vi "Documentation.vi"   [LabVIEW 2019, in "Instrument.Framework-Template.lvclass"]
uses:
  Instrument.Framework-Template.lvclass
  643cabf3-11e0-466e-85d6-f585accee3b6.vi
  bb10f022-7853-4ddd-8dc0-eb6526ad0f54.vi
  61dfef3a-8a93-4f93-91d7-c0ad557d8145.vi
  61dfef3a-8a93-4f93-91d7-c0ad557d8145.vi/a0289200-95e1-4249-98a2-0a47764017b7.vi
  61dfef3a-8a93-4f93-91d7-c0ad557d8145.vi/ef93eee4-b3f8-407d-be7e-7b70ab04c88e.vi
  <vilib>/Utility/Data Type/Get Numeric Information.vi
  <userlib>/LevyLab/Instrument Framework/Instrument/API/Instrument.sendMessageToProcess (string).vi
  <vilib>/Utility/Data Type/Get Type Information.vi
  <vilib>/JDP Science/JSONtext/JSON text to Variant.vi
  <userlib>/LevyLab/Instrument Framework/Instrument/Instrument.lvclass
  <vilib>/JKI/JKI SMO/SMO/SMO.lvclass
  <userlib>/LevyLab/Instrument Framework/Instrument/Typedefs/Instrument.ProtectedCommands--Enum.ctl
  Typedefs/Instrument.Framework-Template.PublicCommands--Enum.ctl
  <userlib>/LevyLab/Instrument Framework/Instrument/Typedefs/Instrument.Commands--Enum.ctl
  Typedefs/Instrument.Framework-Template.getAll--Cluster.ctl
  Typedefs/Instrument.Framework-Template.Configuration--Cluster.ctl
  Typedefs/Instrument.Framework-Template.ProtectedCommands--Enum.ctl
  <vilib>/JDP Science/JSONtext/LVClass Serializer/JSONtext LVClass Serializer.lvclass
  Instrument UI.Framework-Template/Instrument UI.Framework-Template.lvclass
  Instrument UI.Framework-Template/Instrument UI.Framework-Template.UI--Cluster.ctl
  <userlib>/LevyLab/Instrument Framework/Instrument Types/Amplifier/Instrument.Amplifier.lvclass
  <userlib>/LevyLab/Instrument Framework/Instrument Types/CBridge/Instrument.CBridge.lvclass
  <userlib>/LevyLab/Instrument Framework/Instrument Types/Cryostat/Instrument.Cryostat.lvclass
  <userlib>/LevyLab/Instrument Framework/Instrument Types/Delay Line/Instrument.DelayLine.lvclass
  <userlib>/LevyLab/Instrument Framework/Instrument Types/Lockin/Instrument.LockinAPI.lvclass
  <userlib>/LevyLab/Instrument Framework/Instrument Types/Strain/Instrument.Strain.lvclass
  <userlib>/LevyLab/Instrument Framework/Instrument Types/VNA/Instrument.VNA.lvclass
  <userlib>/LevyLab/Instrument Framework/Instrument Types/SCPI/Instrument.SCPI.lvclass
  <userlib>/LevyLab/Instrument Framework/Instrument Types/SignalGenerator/Instrument.SignalGenerator.lvclass
  <userlib>/LevyLab/Instrument Framework/Instrument Types/VSource/Instrument.VSource.lvclass
  <userlib>/LevyLab/Instrument Framework/Instrument UI/Instrument UI.lvclass
  <vilib>/JKI/JKI SMO/SMO.UI/SMO.UI.lvclass
  C:/Program Files (x86)/National Instruments/LabVIEW 2019/user.lib/LevyLab/Instrument Framework/Instrument Types/SCPI/Instrument.SCPI.lvclass
  C:/Program Files (x86)/National Instruments/LabVIEW 2019/user.lib/LevyLab/Instrument Framework/Instrument/Instrument.lvclass
  C:/Program Files (x86)/National Instruments/LabVIEW 2019/vi.lib/JKI/JKI SMO/SMO/SMO.lvclass
  C:/Program Files (x86)/National Instruments/LabVIEW 2019/user.lib/LevyLab/Instrument Framework/Instrument UI/Instrument UI.lvclass
  C:/Program Files (x86)/National Instruments/LabVIEW 2019/vi.lib/JKI/JKI SMO/SMO.UI/SMO.UI.lvclass
types:
  T1 = typedef "Instrument.Framework-Template.lvclass/Instrument.Framework-Template.Configuration--Cluster.ctl" = cluster{"Example Setting 1":dbl, "Example Setting 2":dbl, "Example Setting 3":string}
  T2 = typedef "Instrument.Framework-Template.lvclass/Instrument.Framework-Template.getAll--Cluster.ctl" = cluster{"Levy 1":dbl, "Logger SMO":dbl, "SMO Boolean":bool, "SMO String":string}
  T3 = typedef "Instrument.Framework-Template.lvclass/Instrument.Framework-Template.ProtectedCommands--Enum.ctl" = enum16{"doProtected"}
  T4 = typedef "Instrument.Framework-Template.lvclass/Instrument.Framework-Template.PublicCommands--Enum.ctl" = enum16{"doSomething"}
  T5 = typedef "Instrument.lvclass/Instrument.Commands--Enum.ctl" = enum16{"ACK", "HELP", "IDN", "getAll", "getAllData"}
  T6 = typedef "Instrument.lvclass/Instrument.ProtectedCommands--Enum.ctl" = enum16{"setConfiguration", "setLogData", "setIDN", "setAll", "setAllData"}
  T7 = typedef "Instrument UI.Framework-Template.lvclass/Instrument UI.Framework-Template.UI--Cluster.ctl" = cluster{"Parameter":dbl, "Parameter 2":string}
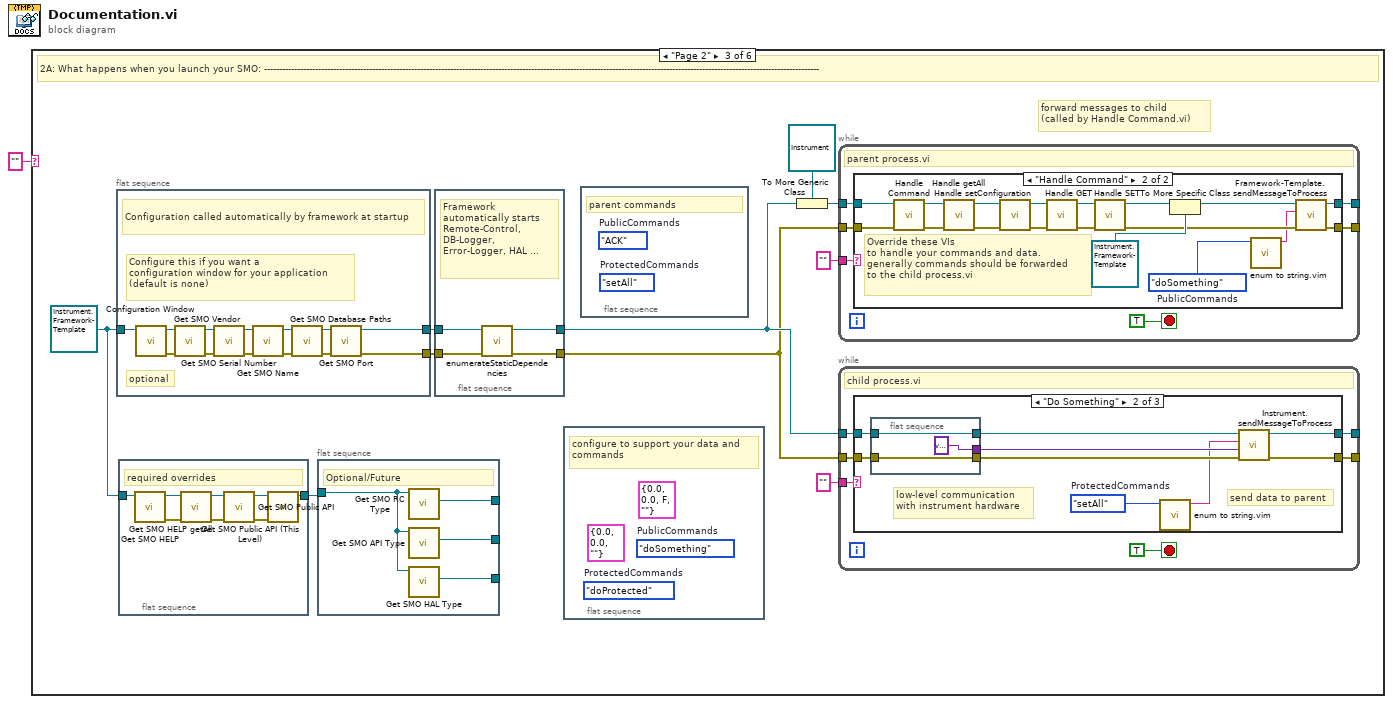
[diagram p0: block diagram]
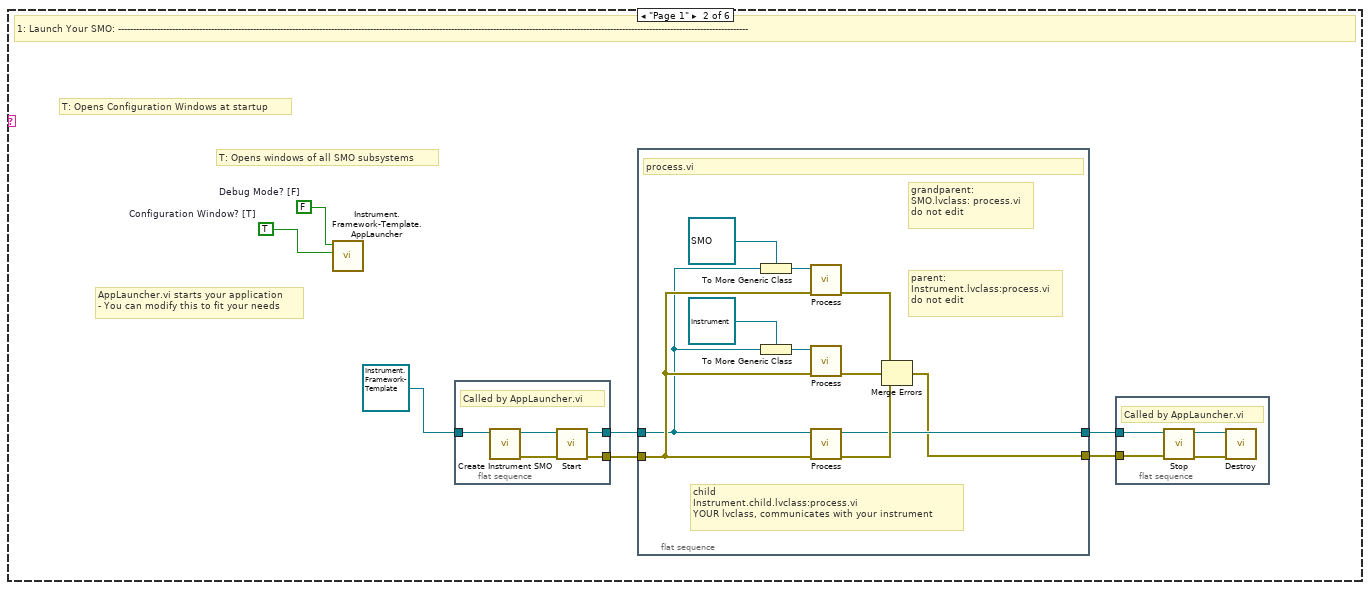
[diagram p3: hidden frame]
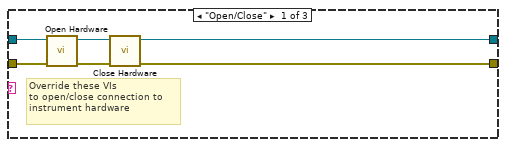
[diagram p4: hidden frame]
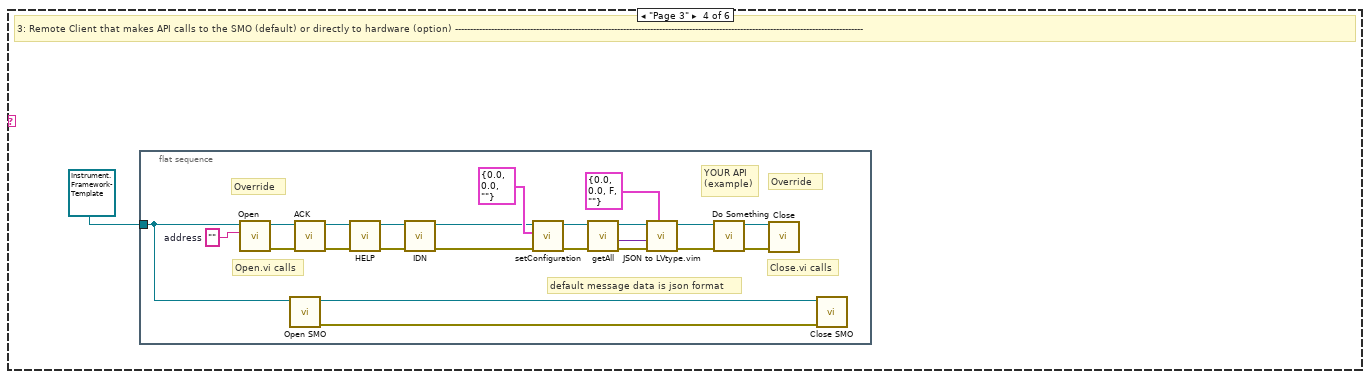
[diagram p7: hidden frame]
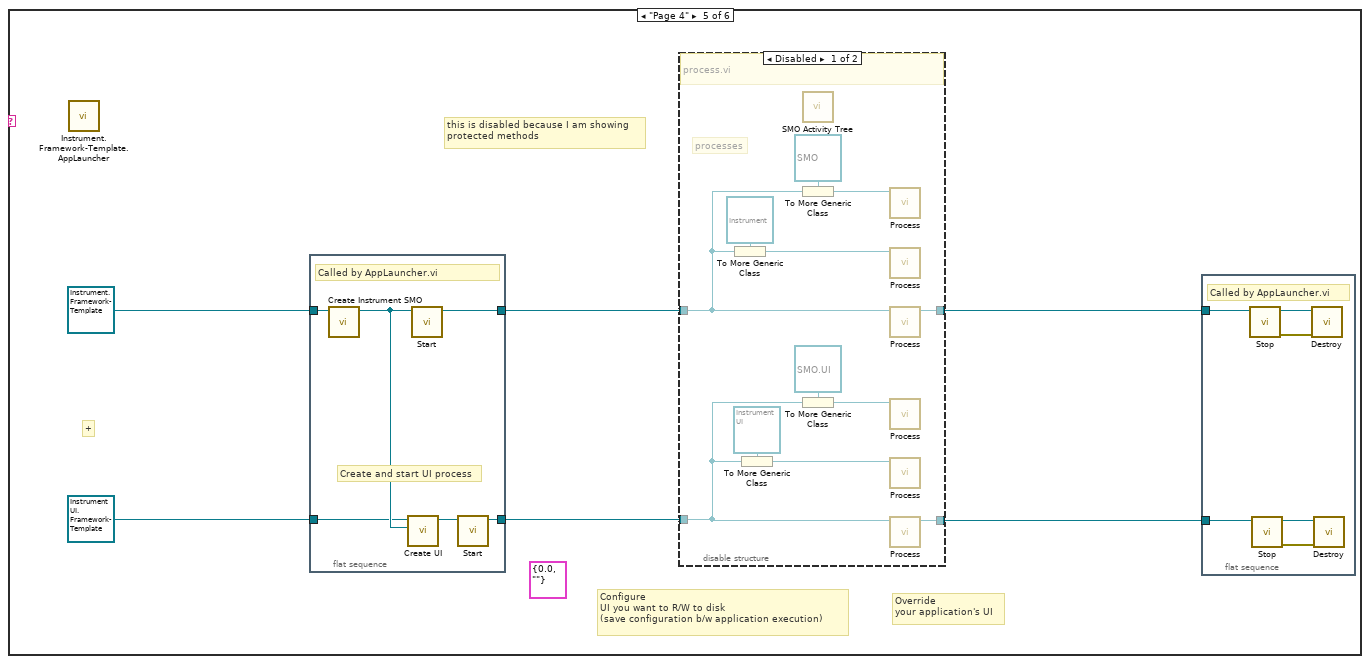
[diagram p8: hidden frame]
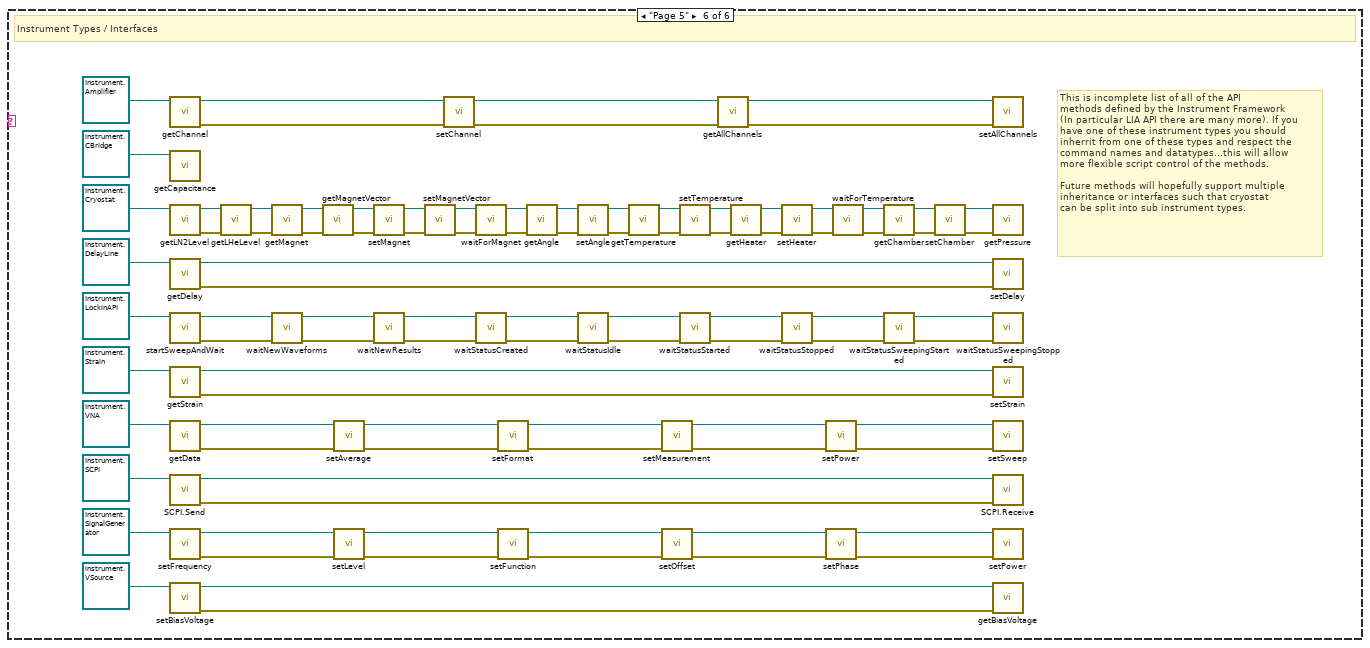
[diagram p10: hidden frame]
diagram:
  n1 = case shown="\"Page 2\"" "" {
    frame Default {
    }
    frame "Page 1" {
      w7 = TRUE  # Configuration Window? [T]
      w8 = FALSE  # Debug Mode? [F]
      # "AppLauncher.vi starts your application\n- You can modify this to fit your needs"
      # "T: Opens windows of all SMO subsystems"
      # "T: Opens Configuration Windows at startup"
      # "1: Launch Your SMO: ------------------------------------------------------------------------------------------------------------------------------------------------------------------------------------------------------------------"
      n2 = call "Instrument.Framework-Template.AppLauncher.vi"("Config Window"=w7, "Debug Mode"=w8) -> ()  [unwired: 9 in, 1 out]
      n3 = flat-sequence {
        tunnel: [w26] -> w3
        tunnel: [w25] -> w5
        tunnel: refnum<class "Instrument.Framework-Template.lvclass"> refnum ("Instrument.Template.lvclass") -> [w24]
        frame #0 {
          # "Called by AppLauncher.vi"
          n4 = call <userlib>:"Create Instrument SMO.vi"("Instrument in"=w24) -> ("error out"=w27:errorcluster, "Instrument out"=w28:refnum<class "Instrument.Framework-Template.lvclass">)  [unwired: 9 in]
          n5 = call <vilib>:"Start.vi"("error in (no error)"=w27, "SMO"=w28) -> ("error out"=w25:errorcluster, "SMO out"=w26:refnum<class "Instrument.Framework-Template.lvclass">)  [unwired: 8 in]
        }
      }
      n6 = flat-sequence {
        tunnel: [w10] -> w6
        tunnel: w5 -> [w18]
        tunnel: [w13] -> w4
        tunnel: w3 -> [w12]
        frame #0 {
          # "child\nInstrument.child.lvclass:process.vi\nYOUR lvclass, communicates with your instrument"
          # "grandparent:\nSMO.lvclass: process.vi\ndo not edit"
          # "parent:\nInstrument.lvclass:process.vi\ndo not edit"
          # "process.vi"
          n7 = To More Generic Class(target class=refnum<class "SMO.lvclass"> refnum ("SMO"), reference=w12) -> (generic class reference=w19:refnum<class "SMO.lvclass">)
          n8 = To More Generic Class(target class=refnum<class "Instrument.lvclass"> refnum ("Instrument"), reference=w12) -> (generic class reference=w17:refnum<class "Instrument.lvclass">)
          n9 = call-dynamic "Process.vi"("error in"=w18, "SMO"=w19) -> ("error out"=w14:errorcluster)  [unwired: 8 in, 1 out]
          n10 = call-dynamic "Process.vi"("error in"=w18, "Instrument"=w17) -> ("error out"=w16:errorcluster)  [unwired: 8 in, 1 out]
          n11 = call-dynamic "Process.vi"("error in"=w18, "Instrument.Framework-Template in"=w12) -> ("error out"=w15:errorcluster, "Instrument.Framework-Template out"=w13:refnum<class "Instrument.Framework-Template.lvclass">)  [unwired: 8 in]
          n12 = Merge Errors(w14, w16, w15) -> (w10:errorcluster)
        }
      }
      n13 = flat-sequence {
        tunnel: w4 -> [w21]
        tunnel: w6 -> [w20]
        frame #0 {
          # "Called by AppLauncher.vi"
          n14 = call <vilib>:"Stop.vi"("error in (no error)"=w20, "SMO"=w21) -> ("error out"=w23:errorcluster, "SMO out"=w22:refnum<class "Instrument.Framework-Template.lvclass">)  [unwired: 8 in]
          n15 = call <vilib>:"Destroy.vi"("error in (no error)"=w23, "SMO"=w22) -> ()  [unwired: 9 in, 1 out]
        }
      }
    }
    frame "Page 2" {
      w32 = refnum<class "Instrument.Framework-Template.lvclass"> refnum ("Instrument.Template.lvclass")
      # "forward messages to child\n(called by Handle Command.vi)"
      # "2A: What happens when you launch your SMO: -----------------------------------------------------------------------------------------------------------------------------------------------------------------------------------------"
      n16 = flat-sequence {
        tunnel: w32 -> [w61]
        tunnel: [w51] -> w33
        tunnel: [w52] -> w34
        frame #0 {
          # "optional"
          # "Configure this if you want a\nconfiguration window for your application\n(default is none)"
          # "Configuration called automatically by framework at startup"
          n17 = call-dynamic "Configuration Window.vi"("Example Instrument in"=w61) -> ("error out"=w63:errorcluster, "Example Instrument out"=w62:refnum<class "Instrument.Framework-Template.lvclass">)  [unwired: 9 in]
          n18 = call-dynamic "Get SMO Vendor.vi"("error in (no error)"=w63, "Instrument.Framework-Template in"=w62) -> ("error out"=w53:errorcluster, "Instrument.Framework-Template out"=w58:refnum<class "Instrument.Framework-Template.lvclass">)  [unwired: 7 in, 1 out]
          n19 = call-dynamic "Get SMO Serial Number.vi"("error in (no error)"=w53, "Instrument.Framework-Template in"=w58) -> ("error out"=w54:errorcluster, "Instrument.Framework-Template out"=w57:refnum<class "Instrument.Framework-Template.lvclass">)  [unwired: 7 in, 1 out]
          n20 = call-dynamic "Get SMO Name.vi"("error in (no error)"=w54, "Instrument.Framework-Template in"=w57) -> ("error out"=w55:errorcluster, "Instrument.Framework-Template out"=w56:refnum<class "Instrument.Framework-Template.lvclass">)  [unwired: 7 in, 1 out]
          n21 = call-dynamic "Get SMO Database Paths.vi"("error in (no error)"=w55, "Instrument.Framework-Template in"=w56) -> ("error out"=w59:errorcluster, "Instrument.Framework-Template out"=w60:refnum<class "Instrument.Framework-Template.lvclass">)  [unwired: 7 in, 1 out]
          n22 = call-dynamic "Get SMO Port.vi"("error in (no error)"=w59, "Instrument.Framework-Template in"=w60) -> ("error out"=w51:errorcluster, "Instrument.Framework-Template out"=w52:refnum<class "Instrument.Framework-Template.lvclass">)  [unwired: 7 in, 1 out]
        }
      }
      n23 = flat-sequence {
        tunnel: w32 -> [w40]
        tunnel: [w39] -> w31
        frame #0 {
          # "required overrides"
          n24 = call-dynamic "Get SMO HELP.vi"("Instrument.Framework-Template in"=w40) -> ("error out"=w46:errorcluster, "Instrument.Framework-Template out"=w45:refnum<class "Instrument.Framework-Template.lvclass">)  [unwired: 8 in, 1 out]
          n25 = call-dynamic "Get SMO HELP getAll.vi"("error in (no error)"=w46, "Instrument.Framework-Template in"=w45) -> ("error out"=w43:errorcluster, "Instrument.Framework-Template out"=w44:refnum<class "Instrument.Framework-Template.lvclass">)  [unwired: 6 in, 2 out]
          n26 = call-dynamic "Get SMO Public API.vi"("error in (no error)"=w43, "Instrument.Framework-Template in"=w44) -> ("error out"=w42:errorcluster, "Instrument.Framework-Template out"=w41:refnum<class "Instrument.Framework-Template.lvclass">)  [unwired: 7 in, 1 out]
          n27 = call-dynamic "Get SMO Public API (This Level).vi"("error in (no error)"=w42, "Instrument.Framework-Template in"=w41) -> ("Instrument.Framework-Template out"=w39:refnum<class "Instrument.Framework-Template.lvclass">)  [unwired: 7 in, 2 out]
        }
      }
      n28 = flat-sequence {
        tunnel: w31 -> [w67]
        tunnel: [w66] -> _
        tunnel: [w65] -> _
        tunnel: [w64] -> _
        frame #0 {
          # "Optional/Future"
          n29 = call-dynamic "Get SMO RC Type.vi"("Instrument in"=w67) -> ("RemoteControl"=w66:refnum<class "RemoteControl.lvclass">)  [unwired: 8 in, 2 out]
          n30 = call-dynamic "Get SMO API Type.vi"("Instrument in"=w67) -> ("API"=w65:refnum<class "API.lvclass">)  [unwired: 8 in, 2 out]
          n31 = call-dynamic "Get SMO HAL Type.vi"("Instrument in"=w67) -> ("Dependencies.HAL"=w64:refnum<class "HAL.lvclass">)  [unwired: 8 in, 2 out]
        }
      }
      n32 = flat-sequence {
        tunnel: w34 -> [w50]
        tunnel: w33 -> [w49]
        tunnel: [w48] -> w30
        tunnel: [w47] -> w29
        frame #0 {
          # "Framework automatically starts\nRemote-Control, DB-Logger, Error-Logger, HAL ..."
          n33 = call-dynamic "enumerateStaticDependencies.vi"("error in (no error)"=w49, "Instrument"=w50) -> ("error out"=w47:errorcluster, "Instrument out"=w48:refnum<class "Instrument.Framework-Template.lvclass">)  [unwired: 7 in, 1 out]
        }
      }
      n34 = flat-sequence {
        frame #0 {
          (unwired) Instrument.Framework-Template.ProtectedCommands--Enum."doProtected"  # ProtectedCommands
          (unwired) T1 {"Example Setting 1"=0.0, "Example Setting 2"=0.0, "Example Setting 3"=""} ("Configuration")
          (unwired) T2 {"Levy 1"=0.0, "Logger SMO"=0.0, "SMO Boolean"=FALSE, "SMO String"=""} ("getAll")
          (unwired) Instrument.Framework-Template.PublicCommands--Enum."doSomething"  # PublicCommands
          # "configure to support your data and commands"
        }
      }
      n35 = flat-sequence {
        frame #0 {
          (unwired) Instrument.Commands--Enum."ACK"  # PublicCommands
          (unwired) Instrument.ProtectedCommands--Enum."setAll"  # ProtectedCommands
          # "parent commands"
        }
      }
      n36 = To More Generic Class(target class=refnum<class "Instrument.lvclass"> refnum ("Instrument"), reference=w30) -> (generic class reference=w35:refnum<class "Instrument.lvclass">)
      n37 = while {
        tunnel: "" -> [w99]
        tunnel: w35 -> [w97]
        tunnel: [w96] -> _
        tunnel: w29 -> [w95]
        tunnel: [w94] -> _
        stop <- TRUE stop-if-true
        # "parent process.vi"
        n38 = case shown="\"Handle Command\"" w99 {
          tunnel: w97 -> [w101 w119]
          tunnel: [w101 w113] -> w96
          tunnel: w95 -> [w100 w118]
          tunnel: [w100 w112] -> w94
          frame Default {
          }
          frame "Handle Command" {
            w103 = Instrument.Framework-Template.PublicCommands--Enum."doSomething"  # PublicCommands
            # "Override these VIs\nto handle your commands and data.\ngenerally commands should be forwarded\nto the child process.vi"
            n39 = call-dynamic "Handle Command.vi"("error in (no error)"=w118, "Instrument in"=w119) -> ("error out"=w114:errorcluster, "Instrument out"=w117:refnum<class "Instrument.lvclass">)  [unwired: 6 in, 2 out]
            n40 = call-dynamic "Handle getAll.vi"("error in (no error)"=w114, "Instrument in"=w117) -> ("error out"=w115:errorcluster, "Instrument out"=w116:refnum<class "Instrument.lvclass">)  [unwired: 7 in, 1 out]
            n41 = call-dynamic "Handle setConfiguration.vi"("error in (no error)"=w115, "Instrument in"=w116) -> ("error out"=w108:errorcluster, "Instrument out"=w109:refnum<class "Instrument.lvclass">)  [unwired: 8 in]
            n42 = call-dynamic "Handle GET.vi"("error in (no error)"=w108, "Instrument in"=w109) -> ("error out"=w106:errorcluster, "Instrument out"=w107:refnum<class "Instrument.lvclass">)  [unwired: 7 in, 1 out]
            n43 = call-dynamic "Handle SET.vi"("error in (no error)"=w106, "Instrument in"=w107) -> ("error out"=w104:errorcluster, "Instrument out"=w105:refnum<class "Instrument.lvclass">)  [unwired: 7 in, 1 out]
            n44 = To More Specific Class(target class=refnum<class "Instrument.Framework-Template.lvclass"> refnum ("Instrument.Template.lvclass"), reference=w105) -> (specific class reference=w111:refnum<class "Instrument.Framework-Template.lvclass">)  [unwired: 1 in, 1 out]
            n45 = call "enum to string.vim"("enum in"=w103) -> ("string out"=w102:string)  [unwired: 9 in, 1 out]
            n46 = call "Framework-Template.sendMessageToProcess.vi"("error in (no error)"=w104, "Command"=w102, "Instrument.Framework-Template in"=w111) -> ("error out"=w112:errorcluster, "Instrument.Framework-Template out"=w113:refnum<class "Instrument.Framework-Template.lvclass">)  [unwired: 7 in]
          }
        }
      }
      n47 = while {
        tunnel: "" -> [w73]
        tunnel: w30 -> [w71]
        tunnel: [w70] -> _
        tunnel: w29 -> [w69]
        tunnel: [w68] -> _
        stop <- TRUE stop-if-true
        # "child process.vi"
        n48 = case shown="\"Do Something\"" w73 {
          tunnel: w71 -> [w76 w84 w93]
          tunnel: [w75 w88 w93] -> w70
          tunnel: w69 -> [w79 w86 w92]
          tunnel: [w74 w87 w92] -> w68
          frame "Open/Close" {
            # "Override these VIs\nto open/close connection to\ninstrument hardware"
            n49 = call-dynamic "Open Hardware.vi"("error in (no error)"=w79, "Instrument in"=w76) -> ("error out"=w78:errorcluster, "Instrument out"=w77:refnum<class "Instrument.Framework-Template.lvclass">)  [unwired: 8 in]
            n50 = call-dynamic "Close Hardware.vi"("error in (no error)"=w78, "Instrument in"=w77) -> ("error out"=w74:errorcluster, "Instrument out"=w75:refnum<class "Instrument.Framework-Template.lvclass">)  [unwired: 8 in]
          }
          frame "Do Something" {
            w81 = Instrument.ProtectedCommands--Enum."setAll"  # ProtectedCommands
            # "low-level communication\nwith instrument hardware"
            # "send data to parent"
            n51 = flat-sequence {
              tunnel: w86 -> [w91]
              tunnel: [w91] -> w85
              tunnel: w84 -> [w90]
              tunnel: [w90] -> w83
              tunnel: [variant ("Data")] -> w82
              frame #0 {
              }
            }
            n52 = call "enum to string.vim"("enum in"=w81) -> ("string out"=w80:string)  [unwired: 9 in, 1 out]
            n53 = call-poly <userlib>:"Instrument.sendMessageToProcess.vi"("error in (no error)"=w85, "Data"=w82, "Command"=w80, "Instrument"=w83) -> ("error out"=w87:errorcluster, "Instrument out"=w88:refnum<class "Instrument.Framework-Template.lvclass">)  [unwired: 6 in]
          }
          frame Default {
          }
        }
      }
    }
    frame "Page 3" {
      # "3: Remote Client that makes API calls to the SMO (default) or directly to hardware (option) ----------------------------------------------------------------------------------------------------------------------------------------"
      n54 = flat-sequence {
        tunnel: refnum<class "Instrument.Framework-Template.lvclass"> refnum ("Instrument.Template.lvclass") -> [w130]
        frame #0 {
          w133 = ""  # address
          # "default message data is json format"
          # "Close.vi calls"
          # "Open.vi calls"
          # "YOUR API\n(example)"
          # "Override"
          # "Override"
          n55 = call-dynamic "Open.vi"("address"=w133, "Instrument.Framework-Template in"=w130) -> ("error out"=w142:errorcluster, "Instrument.Framework-Template out"=w141:refnum<class "Instrument.Framework-Template.lvclass">)  [unwired: 8 in]
          n56 = call <userlib>:"Open SMO.vi"("Instrument in"=w130) -> ("error out"=w131:errorcluster, "Instrument out"=w132:refnum<class "Instrument.Framework-Template.lvclass">)  [unwired: 9 in]
          n57 = call <userlib>:"ACK.vi"("error in (no error)"=w142, "Instrument in"=w141) -> ("error out"=w140:errorcluster, "Instrument out"=w139:refnum<class "Instrument.Framework-Template.lvclass">)  [unwired: 7 in, 1 out]
          n58 = call <userlib>:"HELP.vi"("error in (no error)"=w140, "Instrument in"=w139) -> ("error out"=w123:errorcluster, "Instrument in"=w124:refnum<class "Instrument.Framework-Template.lvclass">)  [unwired: 7 in, 1 out]
          n59 = call <userlib>:"IDN.vi"("error in (no error)"=w123, "Instrument in"=w124) -> ("error out"=w121:errorcluster, "Instrument in"=w122:refnum<class "Instrument.Framework-Template.lvclass">)  [unwired: 7 in, 1 out]
          n60 = call <userlib>:"setConfiguration.vi"("error in (no error)"=w121, "Configuration"=T1 {"Example Setting 1"=0.0, "Example Setting 2"=0.0, "Example Setting 3"=""}, "Instrument in"=w122) -> ("error out"=w134:errorcluster, "Instrument out"=w135:refnum<class "Instrument.Framework-Template.lvclass">)  [unwired: 7 in]
          n61 = call <userlib>:"getAll.vi"("error in (no error)"=w134, "Instrument in"=w135) -> ("error out"=w129:errorcluster, "getAll"=w125:variant, "Instrument out"=w126:refnum<class "Instrument.Framework-Template.lvclass">)  [unwired: 7 in]
          n62 = call "JSON to LVtype.vim"("type"=T2 {"Levy 1"=0.0, "Logger SMO"=0.0, "SMO Boolean"=FALSE, "SMO String"=""} ("getAll"), "error in (no error)"=w129, "JSON Data in"=w125) -> ("error out"=w127:errorcluster)  [unwired: 7 in, 1 out]
          n63 = call-dynamic "Do Something.vi"("error in (no error)"=w127, "Instrument.Framework-Template in"=w126) -> ("error out"=w137:errorcluster, "Instrument.Framework-Template out"=w138:refnum<class "Instrument.Framework-Template.lvclass">)  [unwired: 8 in]
          n64 = call-dynamic "Close.vi"("error in (no error)"=w137, "Instrument.Framework-Template in"=w138) -> ()  [unwired: 8 in, 2 out]
          n65 = call <userlib>:"Close SMO.vi"("error in (no error)"=w131, "Instrument in"=w132) -> ()  [unwired: 8 in, 2 out]
        }
      }
    }
    frame "Page 4" {
      (unwired) T7 {"Parameter"=0.0, "Parameter 2"=""} ("UI")
      # "this is disabled because I am showing\nprotected methods"
      # "Configure\nUI you want to R/W to disk\n(save configuration b/w application execution)"
      # "Override\nyour application's UI"
      # "+"
      n66 = call "Instrument.Framework-Template.AppLauncher.vi"() -> ()  [unwired: 11 in, 1 out]
      n67 = flat-sequence {
        tunnel: [w160] -> w146
        tunnel: refnum<class "Instrument.Framework-Template.lvclass"> refnum ("Instrument.Template.lvclass") -> [w159]
        tunnel: refnum<class "Instrument UI.Framework-Template.lvclass"> refnum ("Instrument UI.Template.lvclass") -> [w157]
        tunnel: [w155] -> w144
        frame #0 {
          # "Create and start UI process"
          # "Called by AppLauncher.vi"
          n68 = call <userlib>:"Create Instrument SMO.vi"("Instrument in"=w159) -> ("Instrument out"=w158:refnum<class "Instrument.Framework-Template.lvclass">)  [unwired: 9 in, 1 out]
          n69 = call <userlib>:"Create UI.vi"("Instrument in"=w158, "Instrument UI"=w157) -> ("Instrument UI out"=w156:refnum<class "Instrument UI.Framework-Template.lvclass">)  [unwired: 8 in, 1 out]
          n70 = call <vilib>:"Start.vi"("SMO"=w158) -> ("SMO out"=w160:refnum<class "Instrument.Framework-Template.lvclass">)  [unwired: 9 in, 1 out]
          n71 = call <vilib>:"Start.vi"("SMO"=w156) -> ("SMO out"=w155:refnum<class "Instrument UI.Framework-Template.lvclass">)  [unwired: 9 in, 1 out]
        }
      }
      n72 = disable-structure shown="Disabled" {
        disable-tunnel: [w172 w174] -> w147
        disable-tunnel: w146 -> [w171 w174]
        disable-tunnel: w144 -> [w170 w173]
        disable-tunnel: [w169 w173] -> w143
        frame Disabled {
          # "processes"
          # "process.vi"
          n73 = To More Generic Class(target class=refnum<class "Instrument.lvclass"> refnum ("Instrument"), reference=w171) -> (generic class reference=w167:refnum<class "Instrument.lvclass">)
          n74 = To More Generic Class(target class=refnum<class "Instrument UI.lvclass"> refnum ("Instrument UI"), reference=w170) -> (generic class reference=w163:refnum<class "Instrument UI.lvclass">)
          n75 = call <vilib>:"SMO Activity Tree.vi"() -> ()  [unwired: 12 in]
          n76 = To More Generic Class(target class=refnum<class "SMO.lvclass"> refnum ("SMO"), reference=w171) -> (generic class reference=w168:refnum<class "SMO.lvclass">)
          n77 = To More Generic Class(target class=refnum<class "SMO.UI.lvclass"> refnum ("SMO.UI"), reference=w170) -> (generic class reference=w161:refnum<class "SMO.UI.lvclass">)
          n78 = call-dynamic "Process.vi"("SMO"=w168) -> ()  [unwired: 9 in, 2 out]
          n79 = call-dynamic "Process.vi"("Instrument"=w167) -> ()  [unwired: 9 in, 2 out]
          n80 = call-dynamic "Process.vi"("Instrument.Framework-Template in"=w171) -> ("Instrument.Framework-Template out"=w172:refnum<class "Instrument.Framework-Template.lvclass">)  [unwired: 9 in, 1 out]
          n81 = call-dynamic "Process.vi"("SMO.UI"=w161) -> ()  [unwired: 9 in, 2 out]
          n82 = call-dynamic "Process.vi"("Instrument UI in"=w163) -> ()  [unwired: 9 in, 2 out]
          n83 = call-dynamic "Process.vi"("Instrument UI.Framework-Template"=w170) -> ("Instrument UI.Framework-Template out"=w169:refnum<class "Instrument UI.Framework-Template.lvclass">)  [unwired: 9 in, 1 out]
        }
        frame Enabled {
        }
      }
      n84 = flat-sequence {
        tunnel: w147 -> [w152]
        tunnel: w143 -> [w150]
        frame #0 {
          # "Called by AppLauncher.vi"
          n85 = call <vilib>:"Stop.vi"("SMO"=w152) -> ("error out"=w154:errorcluster, "SMO out"=w153:refnum<class "Instrument.Framework-Template.lvclass">)  [unwired: 9 in]
          n86 = call <vilib>:"Stop.vi"("SMO"=w150) -> ("error out"=w151:errorcluster, "SMO out"=w149:refnum<class "Instrument UI.Framework-Template.lvclass">)  [unwired: 9 in]
          n87 = call <vilib>:"Destroy.vi"("error in (no error)"=w154, "SMO"=w153) -> ()  [unwired: 9 in, 1 out]
          n88 = call <vilib>:"Destroy.vi"("error in (no error)"=w151, "SMO"=w149) -> ()  [unwired: 9 in, 1 out]
        }
      }
    }
    frame "Page 5" {
      # "This is incomplete list of all of the API\nmethods defined by the Instrument Framework\n(In particular LIA API there are many more). If you\nhave one of these instrument types you should\ninherrit from one of these types and respect the \ncommand names and datatypes...this will allow\nmore flexible script control of the methods.\n\nFuture methods will hopefully support multiple\ninheritance or interfaces such that cryostat\ncan be split into sub instrument types."
      # "Instrument Types / Interfaces"
      n89 = call-dynamic "getChannel.vi"("Instrument.Amplifier in"=refnum<class "Instrument.Amplifier.lvclass"> refnum ("Instrument.Amplifier.lvclass")) -> ("error out"=w255:errorcluster, "Instrument.Amplifier out"=w256:refnum<class "Instrument.Amplifier.lvclass">)  [unwired: 8 in, 1 out]
      n90 = call-dynamic "getCapacitance.vi"("Instrument.CBridge in"=refnum<class "Instrument.CBridge.lvclass"> refnum ("Instrument.CBridge.lvclass")) -> ()  [unwired: 8 in, 3 out]
      n91 = call-dynamic "getLN2Level.vi"("Instrument.Cryostat in"=refnum<class "Instrument.Cryostat.lvclass"> refnum ("Instrument.Cryostat.lvclass")) -> ("error out"=w249:errorcluster, "Instrument.Cryostat out"=w250:refnum<class "Instrument.Cryostat.lvclass">)  [unwired: 8 in, 1 out]
      n92 = call <userlib>:"getDelay.vi"("Instrument.DelayLine in"=refnum<class "Instrument.DelayLine.lvclass"> refnum ("Instrument.DelayLine.lvclass")) -> ("error out"=w217:errorcluster, "Instrument.DelayLine out"=w218:refnum<class "Instrument.DelayLine.lvclass">)  [unwired: 7 in, 2 out]
      n93 = call-dynamic "startSweepAndWait.vi"("Instrument.LockinAPI in"=refnum<class "Instrument.LockinAPI.lvclass"> refnum ("Instrument.LockinAPI.lvclass")) -> ("error out"=w215:errorcluster, "Instrument.LockinAPI out"=w216:refnum<class "Instrument.LockinAPI.lvclass">)  [unwired: 9 in]
      n94 = call-dynamic "getStrain.vi"("Instrument.Strain in"=refnum<class "Instrument.Strain.lvclass"> refnum ("Instrument.Strain.lvclass")) -> ("error out"=w199:errorcluster, "Instrument.Strain out"=w200:refnum<class "Instrument.Strain.lvclass">)  [unwired: 8 in, 1 out]
      n95 = call-dynamic "getData.vi"("Instrument.VSource in"=refnum<class "Instrument.VNA.lvclass"> refnum ("Instrument.VNA.lvclass")) -> ("error out"=w197:errorcluster, "Instrument.VSource out"=w198:refnum<class "Instrument.VNA.lvclass">)  [unwired: 8 in, 1 out]
      n96 = call-dynamic "SCPI.Send.vi"("Instrument.SCPI in"=refnum<class "Instrument.SCPI.lvclass"> refnum ("Instrument.SCPI.lvclass")) -> ("error out"=w187:errorcluster, "Instrument.SCPI out"=w188:refnum<class "Instrument.SCPI.lvclass">)  [unwired: 9 in]
      n97 = call-dynamic "setFrequency.vi"("Instrument.SignalGenerator in"=refnum<class "Instrument.SignalGenerator.lvclass"> refnum ("Instrument.SignalGenerator.lvclass")) -> ("error out"=w185:errorcluster, "Instrument.SignalGenerator out"=w186:refnum<class "Instrument.SignalGenerator.lvclass">)  [unwired: 9 in]
      n98 = call-dynamic "setBiasVoltage.vi"("Instrument.VSource in"=refnum<class "Instrument.VSource.lvclass"> refnum ("Instrument.VSource.lvclass")) -> ("error out"=w175:errorcluster, "Instrument.VSource out"=w176:refnum<class "Instrument.VSource.lvclass">)  [unwired: 9 in]
      n99 = call-dynamic "getLHeLevel.vi"("error in (no error)"=w249, "Instrument.Cryostat in"=w250) -> ("error out"=w247:errorcluster, "Instrument.Cryostat out"=w248:refnum<class "Instrument.Cryostat.lvclass">)  [unwired: 7 in, 1 out]
      n100 = call-dynamic "getMagnet.vi"("error in (no error)"=w247, "Instrument.Cryostat in"=w248) -> ("error out"=w245:errorcluster, "Instrument.Cryostat out"=w246:refnum<class "Instrument.Cryostat.lvclass">)  [unwired: 5 in, 3 out]
      n101 = call-dynamic "waitNewWaveforms.vi"("error in (no error)"=w215, "Instrument.LockinAPI in"=w216) -> ("error out"=w213:errorcluster, "Instrument.LockinAPI out"=w214:refnum<class "Instrument.LockinAPI.lvclass">)  [unwired: 7 in, 1 out]
      n102 = call-dynamic "getMagnetVector.vi"("error in (no error)"=w245, "Instrument.Cryostat in"=w246) -> ("error out"=w243:errorcluster, "Instrument.Cryostat out"=w244:refnum<class "Instrument.Cryostat.lvclass">)  [unwired: 5 in, 3 out]
      n103 = call-dynamic "setAverage.vi"("error in (no error)"=w197, "Instrument.VSource in"=w198) -> ("error out"=w195:errorcluster, "Instrument.VSource out"=w196:refnum<class "Instrument.VNA.lvclass">)  [unwired: 8 in]
      n104 = call-dynamic "setLevel.vi"("error in (no error)"=w185, "Instrument.SignalGenerator in"=w186) -> ("error out"=w183:errorcluster, "Instrument.SignalGenerator out"=w184:refnum<class "Instrument.SignalGenerator.lvclass">)  [unwired: 8 in]
      n105 = call-dynamic "setMagnet.vi"("error in (no error)"=w243, "Instrument.Cryostat in"=w244) -> ("error out"=w241:errorcluster, "Instrument.Cryostat out"=w242:refnum<class "Instrument.Cryostat.lvclass">)  [unwired: 8 in]
      n106 = call-dynamic "waitNewResults.vi"("error in (no error)"=w213, "Instrument.LockinAPI in"=w214) -> ("error out"=w211:errorcluster, "Instrument.LockinAPI out"=w212:refnum<class "Instrument.LockinAPI.lvclass">)  [unwired: 7 in, 1 out]
      n107 = call-dynamic "setMagnetVector.vi"("error in (no error)"=w241, "Instrument.Cryostat in"=w242) -> ("error out"=w239:errorcluster, "Instrument.Cryostat out"=w240:refnum<class "Instrument.Cryostat.lvclass">)  [unwired: 8 in]
      n108 = call-dynamic "setChannel.vi"("error in (no error)"=w255, "Instrument.Amplifier in"=w256) -> ("error out"=w253:errorcluster, "Instrument.Amplifier out"=w254:refnum<class "Instrument.Amplifier.lvclass">)  [unwired: 8 in]
      n109 = call <userlib>:"waitForMagnet.vi"("error in (no error)"=w239, "Instrument.Cryostat in"=w240) -> ("error out"=w237:errorcluster, "Instrument.Cryostat out"=w238:refnum<class "Instrument.Cryostat.lvclass">)  [unwired: 8 in]
      n110 = call-dynamic "waitStatusCreated.vi"("error in (no error)"=w211, "Instrument.LockinAPI in"=w212) -> ("error out"=w209:errorcluster, "Instrument.LockinAPI out"=w210:refnum<class "Instrument.LockinAPI.lvclass">)  [unwired: 8 in]
      n111 = call-dynamic "setFormat.vi"("error in (no error)"=w195, "Instrument.VSource in"=w196) -> ("error out"=w193:errorcluster, "Instrument.VSource out"=w194:refnum<class "Instrument.VNA.lvclass">)  [unwired: 8 in]
      n112 = call-dynamic "setFunction.vi"("error in (no error)"=w183, "Instrument.SignalGenerator in"=w184) -> ("error out"=w181:errorcluster, "Instrument.SignalGenerator out"=w182:refnum<class "Instrument.SignalGenerator.lvclass">)  [unwired: 8 in]
      n113 = call-dynamic "getAngle.vi"("error in (no error)"=w237, "Instrument.Cryostat in"=w238) -> ("error out"=w235:errorcluster, "Instrument.Cryostat out"=w236:refnum<class "Instrument.Cryostat.lvclass">)  [unwired: 5 in, 3 out]
      n114 = call-dynamic "setAngle.vi"("error in (no error)"=w235, "Instrument.Cryostat in"=w236) -> ("error out"=w233:errorcluster, "Instrument.Cryostat out"=w234:refnum<class "Instrument.Cryostat.lvclass">)  [unwired: 8 in]
      n115 = call-dynamic "waitStatusIdle.vi"("error in (no error)"=w209, "Instrument.LockinAPI in"=w210) -> ("error out"=w207:errorcluster, "Instrument.LockinAPI out"=w208:refnum<class "Instrument.LockinAPI.lvclass">)  [unwired: 8 in]
      n116 = call-dynamic "getTemperature.vi"("error in (no error)"=w233, "Instrument.Cryostat in"=w234) -> ("error out"=w231:errorcluster, "Instrument.Cryostat out"=w232:refnum<class "Instrument.Cryostat.lvclass">)  [unwired: 5 in, 3 out]
      n117 = call-dynamic "setMeasurement.vi"("error in (no error)"=w193, "Instrument.VSource in"=w194) -> ("error out"=w191:errorcluster, "Instrument.VSource out"=w192:refnum<class "Instrument.VNA.lvclass">)  [unwired: 8 in]
      n118 = call-dynamic "setOffset.vi"("error in (no error)"=w181, "Instrument.SignalGenerator in"=w182) -> ("error out"=w179:errorcluster, "Instrument.SignalGenerator out"=w180:refnum<class "Instrument.SignalGenerator.lvclass">)  [unwired: 8 in]
      n119 = call-dynamic "setTemperature.vi"("error in (no error)"=w231, "Instrument.Cryostat in"=w232) -> ("error out"=w229:errorcluster, "Instrument.Cryostat out"=w230:refnum<class "Instrument.Cryostat.lvclass">)  [unwired: 8 in]
      n120 = call-dynamic "waitStatusStarted.vi"("error in (no error)"=w207, "Instrument.LockinAPI in"=w208) -> ("error out"=w205:errorcluster, "Instrument.LockinAPI out"=w206:refnum<class "Instrument.LockinAPI.lvclass">)  [unwired: 8 in]
      n121 = call-dynamic "getAllChannels.vi"("error in (no error)"=w253, "Instrument.Amplifier in"=w254) -> ("error out"=w251:errorcluster, "Instrument.Amplifier out"=w252:refnum<class "Instrument.Amplifier.lvclass">)  [unwired: 7 in, 1 out]
      n122 = call-dynamic "getHeater.vi"("error in (no error)"=w229, "Instrument.Cryostat in"=w230) -> ("error out"=w227:errorcluster, "Instrument.Cryostat out"=w228:refnum<class "Instrument.Cryostat.lvclass">)  [unwired: 6 in, 2 out]
      n123 = call-dynamic "setHeater.vi"("error in (no error)"=w227, "Instrument.Cryostat in"=w228) -> ("error out"=w225:errorcluster, "Instrument.Cryostat out"=w226:refnum<class "Instrument.Cryostat.lvclass">)  [unwired: 8 in]
      n124 = call-dynamic "waitStatusStopped.vi"("error in (no error)"=w205, "Instrument.LockinAPI in"=w206) -> ("error out"=w203:errorcluster, "Instrument.LockinAPI out"=w204:refnum<class "Instrument.LockinAPI.lvclass">)  [unwired: 8 in]
      n125 = call-dynamic "setPower.vi"("error in (no error)"=w191, "Instrument.VSource in"=w192) -> ("error out"=w189:errorcluster, "Instrument.VSource out"=w190:refnum<class "Instrument.VNA.lvclass">)  [unwired: 8 in]
      n126 = call-dynamic "setPhase.vi"("error in (no error)"=w179, "Instrument.SignalGenerator in"=w180) -> ("error out"=w177:errorcluster, "Instrument.SignalGenerator out"=w178:refnum<class "Instrument.SignalGenerator.lvclass">)  [unwired: 8 in]
      n127 = call <userlib>:"waitForTemperature.vi"("error in (no error)"=w225, "Instrument.Cryostat in"=w226) -> ("error out"=w223:errorcluster, "Instrument.Cryostat out"=w224:refnum<class "Instrument.Cryostat.lvclass">)  [unwired: 8 in]
      n128 = call-dynamic "getChamber.vi"("error in (no error)"=w223, "Instrument.Cryostat in"=w224) -> ("error out"=w221:errorcluster, "Instrument.Cryostat out"=w222:refnum<class "Instrument.Cryostat.lvclass">)  [unwired: 7 in, 1 out]
      n129 = call-dynamic "waitStatusSweepingStarted.vi"("error in (no error)"=w203, "Instrument.LockinAPI in"=w204) -> ("error out"=w201:errorcluster, "Instrument.LockinAPI out"=w202:refnum<class "Instrument.LockinAPI.lvclass">)  [unwired: 8 in]
      n130 = call-dynamic "setChamber.vi"("error in (no error)"=w221, "Instrument.Cryostat in"=w222) -> ("error out"=w219:errorcluster, "Instrument.Cryostat out"=w220:refnum<class "Instrument.Cryostat.lvclass">)  [unwired: 8 in]
      n131 = call-dynamic "setAllChannels.vi"("error in (no error)"=w251, "Instrument.Amplifier in"=w252) -> ()  [unwired: 8 in, 2 out]
      n132 = call-dynamic "getPressure.vi"("error in (no error)"=w219, "Instrument.Cryostat in"=w220) -> ()  [unwired: 6 in, 4 out]
      n133 = call-dynamic "setDelay.vi"("error in (no error)"=w217, "Instrument.Delay in"=w218) -> ()  [unwired: 8 in, 2 out]
      n134 = call-dynamic "waitStatusSweepingStopped.vi"("error in (no error)"=w201, "Instrument.LockinAPI in"=w202) -> ()  [unwired: 8 in, 2 out]
      n135 = call-dynamic "setStrain.vi"("error in (no error)"=w199, "Instrument.Strain in"=w200) -> ()  [unwired: 8 in, 2 out]
      n136 = call-dynamic "setSweep.vi"("error in (no error)"=w189, "Instrument.VSource in"=w190) -> ()  [unwired: 8 in, 2 out]
      n137 = call-dynamic "SCPI.Receive.vi"("error in (no error)"=w187, "Instrument.SCPI in"=w188) -> ()  [unwired: 7 in, 3 out]
      n138 = call-dynamic "setPower.vi"("error in (no error)"=w177, "Instrument.SignalGenerator in"=w178) -> ()  [unwired: 8 in, 2 out]
      n139 = call-dynamic "getBiasVoltage.vi"("error in (no error)"=w175, "Instrument.VSource in"=w176) -> ()  [unwired: 7 in, 3 out]
    }
  }
